vi "pco.camera_SaveMean_Example_IMAQ.vi"() -> ()   [LabVIEW 2020]
uses:
  Camera.lvclass
panel:
  out "rawImage":u16[][](array[numeric])
  out "Image":T1(plugin-control)
  in  "data_format":T2(ring)=enum."Mono16"
  in  "Image Index":u32 max=9
  in  "saveImages":bool
  in  "SavePath":path
  out "Recorded Images":u32
  in  "Quit":bool
  in  "roiY1":u64=2 min=2 max=1040 step=1
  in  "roiX1":u64=2 min=2 max=1392 step=1
  in  "roiY0":u64=1 min=1 max=1039 step=1
  in  "roiX0":u64=1 min=1 max=1391 step=1
  out "Image Height":u16
  out "Image Width":u16
  in  "dwImgCount":u32=10 caption="Required Number of Images" max=4023
  out "Error":errorcluster {"code" format="%x"}
  # "This example shows how to record an image sequence, get the mean of that sequence and save it to file afterwards.\nIt is a good starting point for writing own applications.\nBut it will not be fail save, i.e. doesnt react on errors, just handles them forward to the end\n\nUsage:\nSelect your required image count you want to average over before you start the program.\nOnce started, the camera class will be initialized and images will be recorded automatically.\nTWhen acquisition has finished the mean image is read and shown.\nNow you can crop the image using the ROI parameters and select a file path.\nBy clicking save, the mean image is saved with the selected file format using the current roi setting\nThis also finishes the program and will force an exit of the camera class"
  # "pco.labview"
  # "Camera Setup"
  # "Recording Control"
  # "Parameters for image readout"
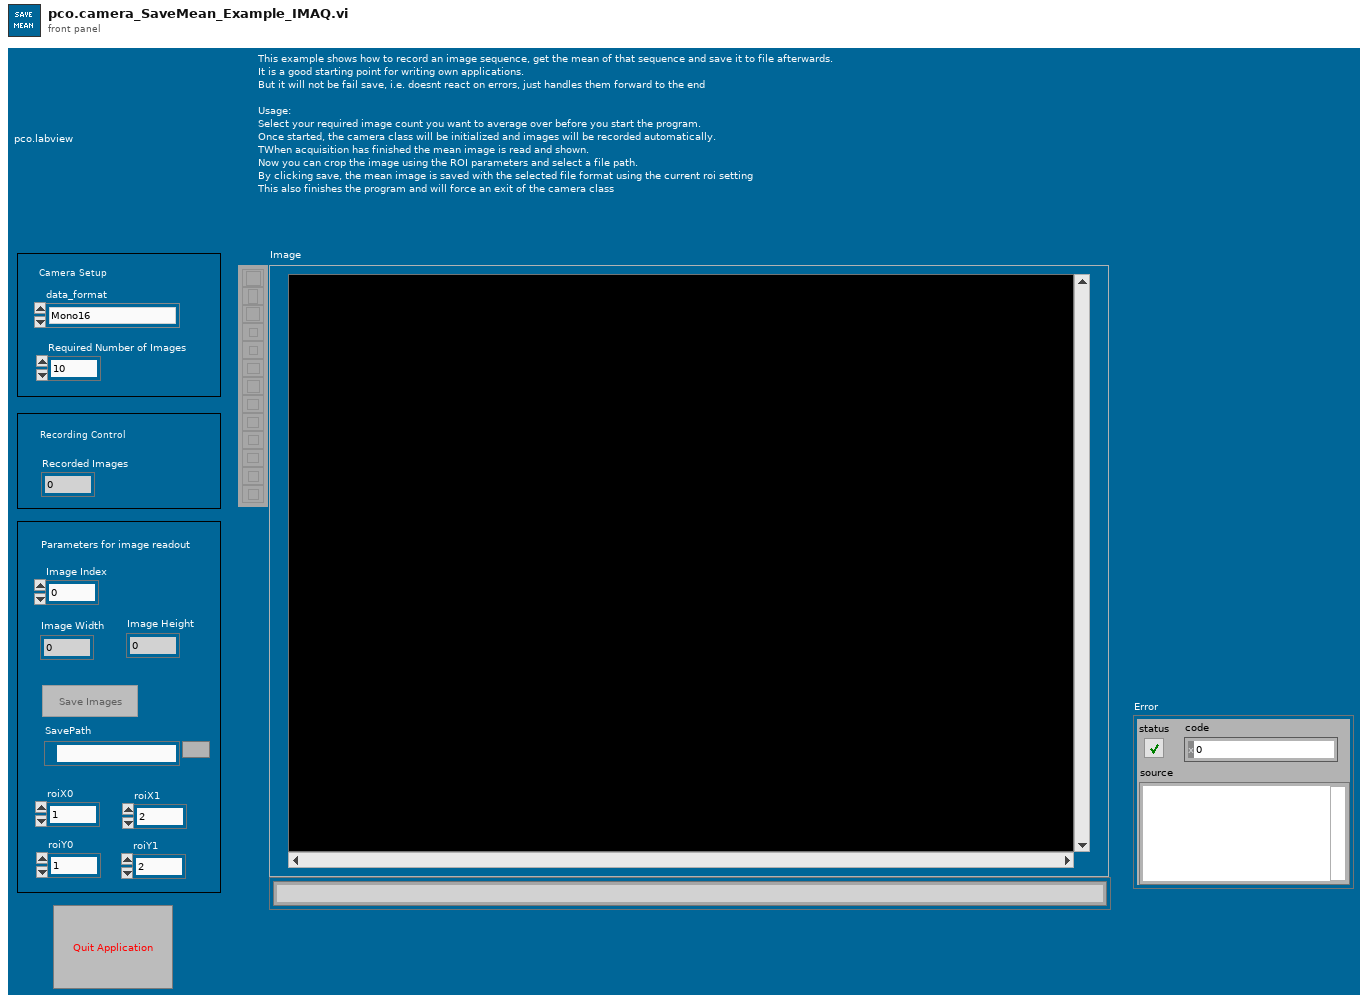
[diagram p1: front panel]
types:
  T1 = typedef "IMAQ Image.ctl" = refnum<image>
  T2 = enum16{"Undefined", "Mono8", "Mono16", "BGRA8", "RGBA8", "BGRA16", "RGBA16", "CompressedMono8"}
  T3 = enum8{"Enabled", "Disabled", "Disabled and Grayed Out"}
  T4 = enum16{"sequence", "sequence non blocking", "ring buffer", "fifo", "sequence_dpcore", "sequence_non_blocking_dpcore", "ring_buffer_dpcore", "fifo_dpcore", "tif", "multitif", "pcoraw", "b16", "dicom", "multidicom"}
  T5 = cluster{"serial":u32, "type":u16, "sub_type":u16, "interface_type":u16, "bit_resolution":u16, "min_exposure_time_s":dbl, "max_exposure_time_s":dbl, "min_exposure_step_s":dbl, "min_delay_time_s":dbl, "max_delay_time_s":dbl, "min_delay_step_s":dbl, "min_width":u64, "min_height":u64, "max_width":u64, "max_height":u64, "roi_step_horz":u64, "roi_step_vert":u64, "roi_symmetric_horz":bool, "roi_symmetric_vert":bool, "has_timestamp_mode":bool, "has_timestamp_mode_ascii_only":bool, "pixelrate_vec":u32[], "has_acquire_mode":bool, "has_ext_acquire_mode":bool, "has_metadata_mode":bool, "has_ram":bool, "binning_horz_vec":u16[], "binning_vert_vec":u16[]}
  T6 = typedef "Image Type" = u32
  T7 = typedef "Camera.lvclass/binning.ctl" = cluster{"vert":u16, "horz":u16}
  T8 = cluster{"exposure_time_s":dbl, "delay_time_s":dbl, "roi":cluster{"x0":u64, "y0":u64, "x1":u64, "y1":u64}, "timestamp_mode":u16, "pixelrate":u32, "trigger_mode":u16, "acquire_mode":u16, "metadata_mode":u16, "noisefilter_mode":u16, "binning":T7}
  T9 = cluster{"Plane 4 (alpha)":u16, "Plane 1 (Red)":u16, "Plane 2 (Green)":u16, "Plane 3 (Blue)":u16}[][]
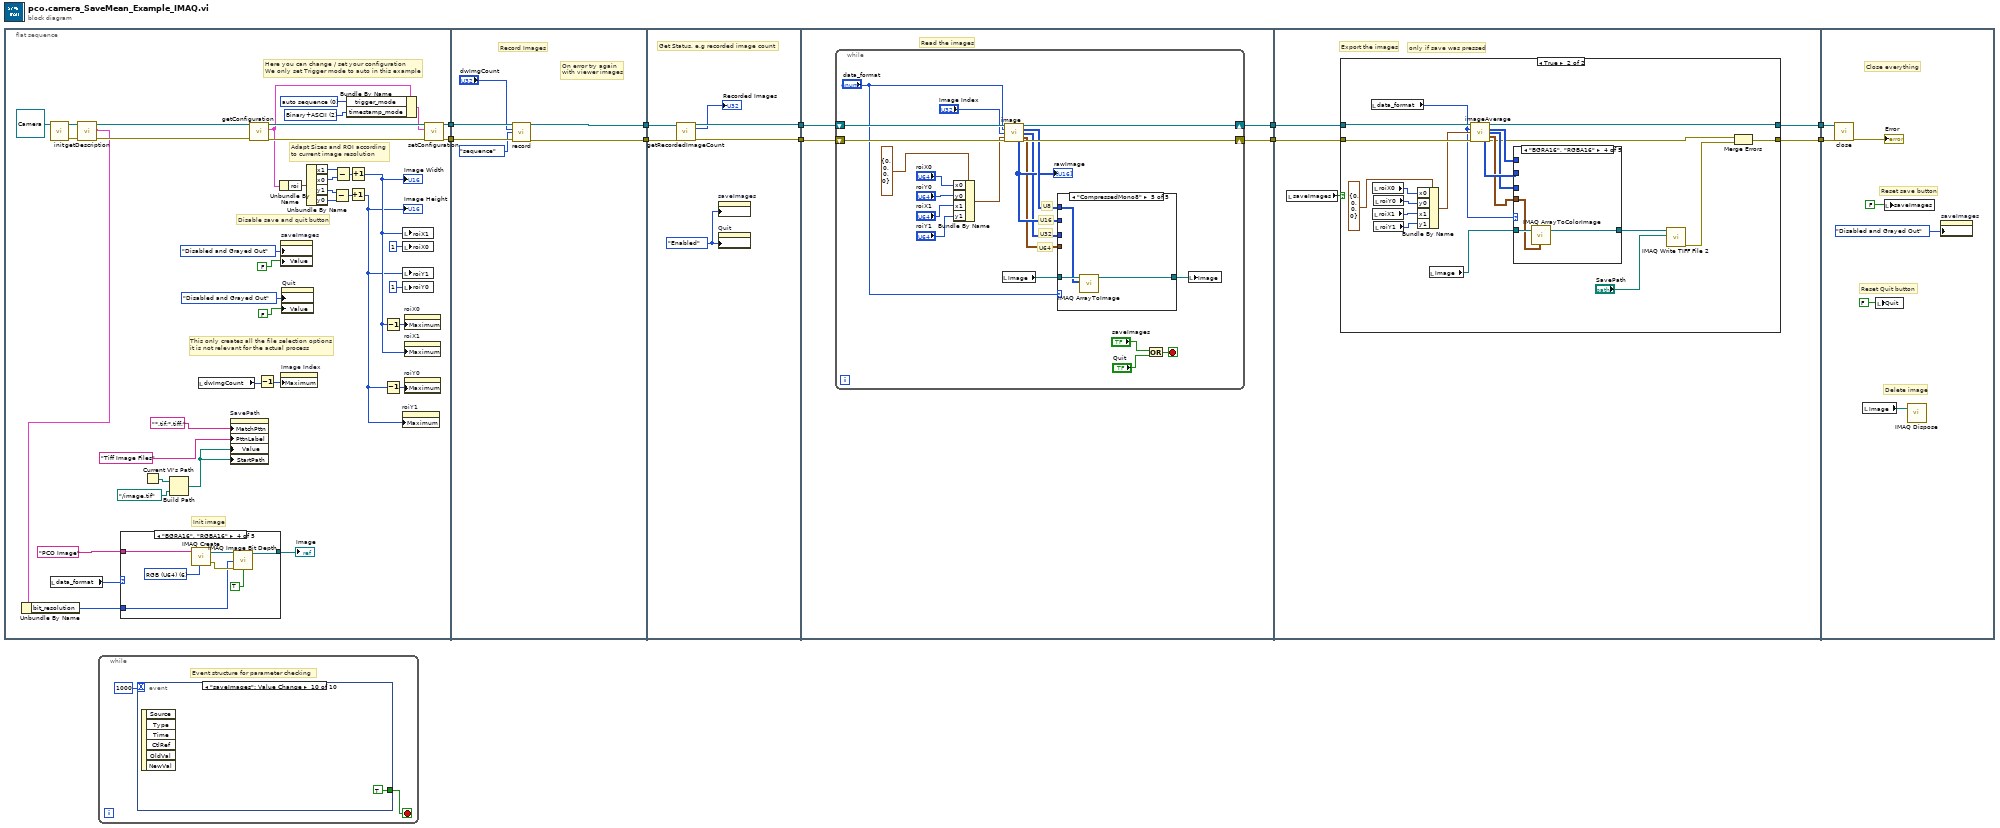
[diagram p0: block diagram]
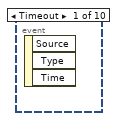
[diagram p2: hidden frame]
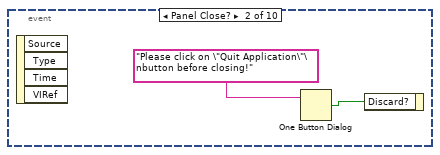
[diagram p3: hidden frame]
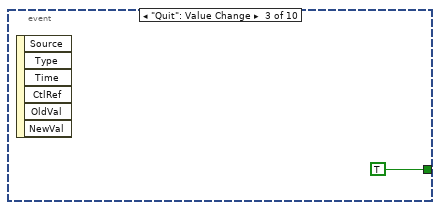
[diagram p4: hidden frame]
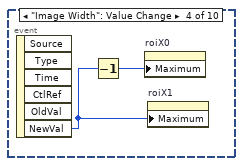
[diagram p5: hidden frame]
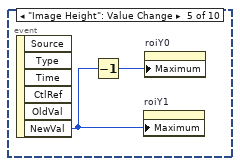
[diagram p6: hidden frame]
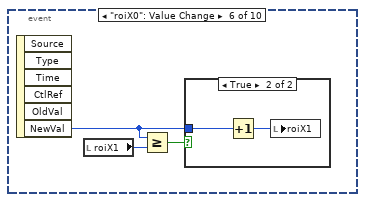
[diagram p7: hidden frame]
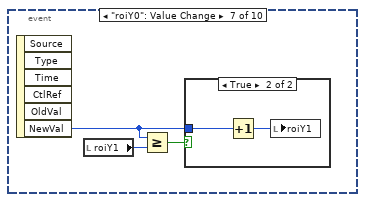
[diagram p9: hidden frame]
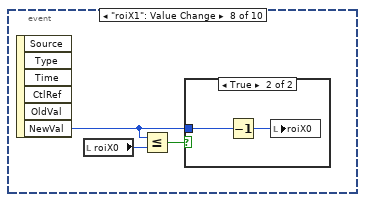
[diagram p11: hidden frame]
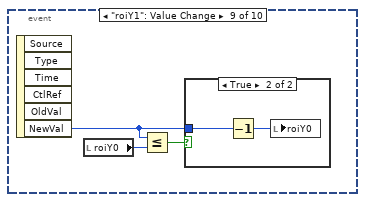
[diagram p13: hidden frame]
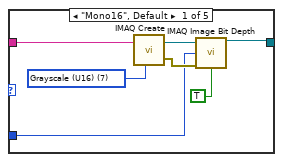
[diagram p15: hidden frame]
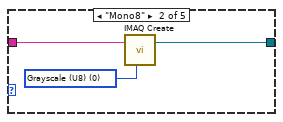
[diagram p16: hidden frame]
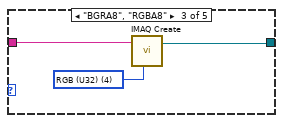
[diagram p17: hidden frame]
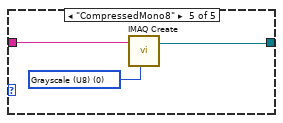
[diagram p18: hidden frame]
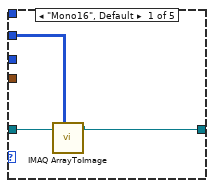
[diagram p19: hidden frame]
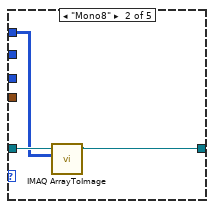
[diagram p20: hidden frame]
diagram:
  n1 = flat-sequence {
    tunnel: [w45] -> w10
    tunnel: [w44] -> w9
    tunnel: w10 -> [w81]
    tunnel: w9 -> [w80]
    tunnel: [w78] -> w8
    tunnel: [w77] -> w7
    tunnel: w8 -> [w87]
    tunnel: w7 -> [w86]
    tunnel: [w85] -> w6
    tunnel: [w84] -> w5
    tunnel: w6 -> [w90]
    tunnel: w5 -> [w91]
    tunnel: [w89] -> w4
    tunnel: [w88] -> w2
    tunnel: w4 -> [w131]
    tunnel: [w130] -> w3
    tunnel: w2 -> [w129]
    tunnel: [w128] -> w1
    tunnel: w3 -> [w176]
    tunnel: w1 -> [w175]
    frame #0 {
      w29 = u16 2 items=["OFF", "Binary", "Binary+ASCII", "ASCII"] ("TimestampMode")
      w51 = u16 0 items=["auto sequence"=0, "software trigger"=1, "external exposure start & software trigger"=2, "external exposure control"=3, "external synchronized"=4, "fast external exposure control"=5, "external CDS control"=6, "slow external exposure control"=7, "external synchronized HDSDI"=258] ("TriggerMode")
      # "Init image"
      # "This only creates all the file selection options\nit is not relevant for the actual process"
      # "Adapt Sizes and ROI according\nto current image resolution"
      # "Disable save and quit button"
      # "Here you can change / set your configuration\nWe only set Trigger mode to auto in this example"
      n2 = call-dynamic "init.vi"("Camera in"=refnum<class "Camera.lvclass"> refnum ("PCOCamera in")) -> ("Camera out"=w15:refnum<class "Camera.lvclass">, "error out"=w16:errorcluster)  [unwired: 8 in]
      n3 = local read "data_format"() -> (w19:T2)
      n4 = call-dynamic "getDescription.vi"("error in (no error)"=w16, "Camera in"=w15) -> ("error out"=w13:errorcluster, "description"=w12:T5, "Camera out"=w14:refnum<class "Camera.lvclass">)  [unwired: 7 in]
      n5 = Unbundle By Name(w12) -> ("bit_resolution"=w11:u16)
      n6 = case shown="\"BGRA16\", \"RGBA16\"" w19 {
        tunnel: "PCO Image" ("Image Name") -> [w58 w62 w64 w71 w74]
        tunnel: [w54 w60 w63 w68 w73] -> w18
        tunnel: w11 -> [w53 _ _ w66 _]
        frame "Mono16", Default {
          w59 = T6 7 items=["Grayscale (U8)", "Grayscale (I16)", "Grayscale (SGL)", "Complex (CSG)", "RGB (U32)", "HSL (U32)", "RGB (U64)", "Grayscale (U16)"] ("Image Type")
          n7 = call "IMAQ Create"("Image Name"=w58, "Image Type"=w59) -> ("New Image"=w56:T1, "error out"=w55:errorcluster)  [unwired: 3 in]
          n8 = call "IMAQ Image Bit Depth"("Image"=w56, "Bit Depth (0)"=w53, "error in (no error)"=w55, "Get/Set Bit Depth? (Set)"=TRUE) -> ("Image Out"=w54:T1)  [unwired: 9 in, 2 out]
        }
        frame "Mono8" {
          w61 = T6 0 items=["Grayscale (U8)", "Grayscale (I16)", "Grayscale (SGL)", "Complex (CSG)", "RGB (U32)", "HSL (U32)", "RGB (U64)", "Grayscale (U16)"] ("Image Type")
          n9 = call "IMAQ Create"("Image Name"=w62, "Image Type"=w61) -> ("New Image"=w60:T1)  [unwired: 3 in, 1 out]
        }
        frame "BGRA8", "RGBA8" {
          w65 = T6 4 items=["Grayscale (U8)", "Grayscale (I16)", "Grayscale (SGL)", "Complex (CSG)", "RGB (U32)", "HSL (U32)", "RGB (U64)", "Grayscale (U16)"] ("Image Type")
          n10 = call "IMAQ Create"("Image Name"=w64, "Image Type"=w65) -> ("New Image"=w63:T1)  [unwired: 3 in, 1 out]
        }
        frame "BGRA16", "RGBA16" {
          w72 = T6 6 items=["Grayscale (U8)", "Grayscale (I16)", "Grayscale (SGL)", "Complex (CSG)", "RGB (U32)", "HSL (U32)", "RGB (U64)", "Grayscale (U16)"] ("Image Type")
          n11 = call "IMAQ Create"("Image Name"=w71, "Image Type"=w72) -> ("New Image"=w69:T1, "error out"=w67:errorcluster)  [unwired: 3 in]
          n12 = call "IMAQ Image Bit Depth"("Image"=w69, "Bit Depth (0)"=w66, "error in (no error)"=w67, "Get/Set Bit Depth? (Set)"=TRUE) -> ("Image Out"=w68:T1)  [unwired: 9 in, 2 out]
        }
        frame "CompressedMono8" {
          w75 = T6 0 items=["Grayscale (U8)", "Grayscale (I16)", "Grayscale (SGL)", "Complex (CSG)", "RGB (U32)", "HSL (U32)", "RGB (U64)", "Grayscale (U16)"] ("Image Type")
          n13 = call "IMAQ Create"("Image Name"=w74, "Image Type"=w75) -> ("New Image"=w73:T1)  [unwired: 3 in, 1 out]
        }
      }
      "Image" <- w18
      n14 = Current VI's Path() -> (path=w26:path)
      n15 = Build Path(base path=w26, name or relative path=path "../image.tif" ("SavePath")) -> (appended path=w23:path)
      n16 = local read "dwImgCount"() -> (w21:u32)
      n17 = property on="SavePath" class="Path"("MatchPttn"="*.tif;*.tiff;" ("pattern (all files)"), "PttnLabel"="Tiff Image Files" ("pattern label"), "Value"=w23, "StartPath"=w23) -> ()  [unwired: 2 in, 2 out]
      n18 = call-dynamic "getConfiguration.vi"("error in (no error)"=w13, "Camera in"=w14) -> ("error out"=w49:errorcluster, "configuration"=w39:T8, "Camera out"=w50:refnum<class "Camera.lvclass">)  [unwired: 7 in]
      n19 = Decrement(x=w21) -> (x-1=w22:u32)
      n20 = Unbundle By Name(w39) -> ("roi"=w38:cluster{"x0":u64, "y0":u64, "x1":u64, "y1":u64})
      n21 = property on="saveImages" class="Bool (strict)"("DisabledEnum"=T3."Disabled and Grayed Out" ("Disabled"), "Value"=FALSE ("Stop")) -> ()  [unwired: 2 in, 2 out]
      n22 = property on="Image Index" class="DigNum (strict)"("Maximum"=w22) -> ()  [unwired: 2 in, 2 out]
      n23 = property on="Quit" class="Bool (strict)"("DisabledEnum"=T3."Disabled and Grayed Out" ("Disabled"), "Value"=FALSE ("Stop")) -> ()  [unwired: 2 in, 2 out]
      n24 = Unbundle By Name(w38) -> ("x1"=w36:u64, "x0"=w37:u64, "y1"=w34:u64, "y0"=w35:u64)
      n25 = Subtract(x=w34, y=w35) -> (x-y=w32:u64)
      n26 = Subtract(x=w36, y=w37) -> (x-y=w33:u64)
      n27 = Bundle By Name(cluster=w39, "trigger_mode"=w51, "timestamp_mode"=w29) -> (w48:T8)
      n28 = Increment(x=w32) -> (x+1=w30:u64)
      "Image Height" <- w30
      n29 = Increment(x=w33) -> (x+1=w31:u64)
      "Image Width" <- w31
      n30 = Decrement(x=w31) -> (x-1=w41:u64)
      n31 = Decrement(x=w30) -> (x-1=w40:u64)
      n32 = property on="roiY1" class="DigNum (strict)"("Maximum"=w30) -> ()  [unwired: 2 in, 2 out]
      n33 = local write "roiX1"(w31) -> ()
      n34 = local write "roiX0"(u16 1 ("roiY0")) -> ()
      n35 = local write "roiY1"(w30) -> ()
      n36 = local write "roiY0"(u16 1 ("roiY0")) -> ()
      n37 = property on="roiX0" class="DigNum (strict)"("Maximum"=w41) -> ()  [unwired: 2 in, 2 out]
      n38 = property on="roiX1" class="DigNum (strict)"("Maximum"=w31) -> ()  [unwired: 2 in, 2 out]
      n39 = property on="roiY0" class="DigNum (strict)"("Maximum"=w40) -> ()  [unwired: 2 in, 2 out]
      n40 = call-dynamic "setConfiguration.vi"("error in (no error)"=w49, "configuration"=w48, "Camera in"=w50) -> ("error out"=w44:errorcluster, "Camera out"=w45:refnum<class "Camera.lvclass">)  [unwired: 7 in]
    }
    frame #1 {
      # "On error try again \nwith viewer images"
      # "Record Images"
      n41 = call-dynamic "record.vi"("Camera in"=w81, "num_images"="dwImgCount", "record_mode"=T4."sequence", "error in (no error)"=w80) -> ("Camera out"=w78:refnum<class "Camera.lvclass">, "error out"=w77:errorcluster)  [unwired: 10 in]
    }
    frame #2 {
      w82 = T3."Enabled" ("Disabled")
      # "Get Status, e.g recorded image count"
      n42 = call-dynamic "getRecordedImageCount.vi"("Camera in"=w87, "error in (no error)"=w86) -> ("Camera out"=w85:refnum<class "Camera.lvclass">, "recorded_image_count"=→"Recorded Images":u32, "error out"=w84:errorcluster)  [unwired: 11 in]
      n43 = property on="saveImages" class="Bool (strict)"("DisabledEnum"=w82) -> ()  [unwired: 2 in, 2 out]
      n44 = property on="Quit" class="Bool (strict)"("DisabledEnum"=w82) -> ()  [unwired: 2 in, 2 out]
    }
    frame #3 {
      # "Read the images"
      n45 = while {
        shift-right: [w110] -> w89
        shift-left: w90 -> [w112]
        shift-right: [w105] -> w88
        shift-left: w91 -> [w111]
        stop <- w103 stop-if-true
        # "U64"
        # "U32"
        # "U16"
        # "U8"
        n46 = Bundle By Name(cluster=cluster{"x0":u64, "y0":u64, "x1":u64, "y1":u64} {"x0"=0, "y0"=0, "x1"=0, "y1"=0} ("roi"), "x0"="roiX0", "y0"="roiY0", "x1"="roiX1", "y1"="roiY1") -> (w101:cluster{"x0":u64, "y0":u64, "x1":u64, "y1":u64})
        n47 = local read "Image"() -> (w94:T1)
        n48 = call-dynamic "image.vi"("Camera in"=w112, "data_format"="data_format", "image_index"="Image Index", "roi"=w101, "error in (no error)"=w111) -> ("Camera out"=w110:refnum<class "Camera.lvclass">, "image (U8)"=w98:u8[][], "image (U32)"=w96:u32[][], "image (U64)"=w95:T9, "raw_image (U16)"=w97:u16[][], "error out"=w105:errorcluster)  [unwired: 3 in, 2 out]
        "rawImage" <- w97
        n49 = case shown="\"CompressedMono8\"" "data_format" {
          tunnel: w94 -> [w115 w118 w121 w124 w127]
          tunnel: [w113 w116 w120 w122 w126] -> w93
          tunnel: w95 -> [_ _ _ w123 _]
          tunnel: w96 -> [_ _ w119 _ _]
          tunnel: w98 -> [_ w117 _ _ w125]
          tunnel: w97 -> [w114 _ _ _ _]
          frame "Mono16", Default {
            n50 = call "IMAQ ArrayToImage"("Image Pixels (U16)"=w114, "Image"=w115) -> ("Image Out"=w113:T1)  [unwired: 8 in, 1 out]
          }
          frame "Mono8" {
            n51 = call "IMAQ ArrayToImage"("Image Pixels (U8)"=w117, "Image"=w118) -> ("Image Out"=w116:T1)  [unwired: 8 in, 1 out]
          }
          frame "BGRA8", "RGBA8" {
            n52 = call "IMAQ ArrayToColorImage"("Image Pixels (U32)"=w119, "Image"=w121) -> ("Image Out"=w120:T1)  [unwired: 3 in, 1 out]
          }
          frame "BGRA16", "RGBA16" {
            n53 = call "IMAQ ArrayToColorImage"("Image"=w124, "Image Pixels (U64)"=w123) -> ("Image Out"=w122:T1)  [unwired: 3 in, 1 out]
          }
          frame "CompressedMono8" {
            n54 = call "IMAQ ArrayToImage"("Image Pixels (U8)"=w125, "Image"=w127) -> ("Image Out"=w126:T1)  [unwired: 8 in, 1 out]
          }
        }
        n55 = Or(x="saveImages", y="Quit") -> (x .or. y?=w103:bool)
        n56 = local write "Image"(w93) -> ()
      }
    }
    frame #4 {
      # "only if save was pressed"
      # "Export the images"
      n57 = local read "saveImages"() -> (w132:bool)
      n58 = case shown="True" w132 {
        tunnel: w131 -> [w134 w153]
        tunnel: [w134 w142] -> w130
        tunnel: w129 -> [w133 w154]
        tunnel: [w133 w140] -> w128
        frame False {
        }
        frame True {
          n59 = local read "data_format"() -> (w138:T2)
          n60 = local read "roiX0"() -> (w151:u64)
          n61 = local read "roiX1"() -> (w149:u64)
          n62 = local read "roiY0"() -> (w150:u64)
          n63 = local read "roiY1"() -> (w148:u64)
          n64 = Bundle By Name(cluster=cluster{"x0":u64, "y0":u64, "x1":u64, "y1":u64} {"x0"=0, "y0"=0, "x1"=0, "y1"=0} ("roi"), "x0"=w151, "y0"=w150, "x1"=w149, "y1"=w148) -> (w147:cluster{"x0":u64, "y0":u64, "x1":u64, "y1":u64})
          n65 = local read "Image"() -> (w139:T1)
          n66 = call-dynamic "imageAverage.vi"("Camera in"=w153, "data_format"=w138, "roi"=w147, "error in (no error)"=w154) -> ("Camera out"=w142:refnum<class "Camera.lvclass">, "image (U8)"=w146:u8[][], "image (U32)"=w144:u32[][], "image (U64)"=w143:T9, "raw_image (U16)"=w145:u16[][], "error out"=w141:errorcluster)  [unwired: 6 in]
          n67 = case shown="\"BGRA16\", \"RGBA16\"" w138 {
            tunnel: w139 -> [w157 w160 w163 w166 w169]
            tunnel: [w155 w158 w162 w164 w168] -> w136
            tunnel: w143 -> [_ _ _ w165 _]
            tunnel: w144 -> [_ _ w161 _ _]
            tunnel: w146 -> [_ w159 _ _ w167]
            tunnel: w145 -> [w156 _ _ _ _]
            frame "Mono16", Default {
              n68 = call "IMAQ ArrayToImage"("Image Pixels (U16)"=w156, "Image"=w157) -> ("Image Out"=w155:T1)  [unwired: 8 in, 1 out]
            }
            frame "Mono8" {
              n69 = call "IMAQ ArrayToImage"("Image Pixels (U8)"=w159, "Image"=w160) -> ("Image Out"=w158:T1)  [unwired: 8 in, 1 out]
            }
            frame "BGRA8", "RGBA8" {
              n70 = call "IMAQ ArrayToColorImage"("Image Pixels (U32)"=w161, "Image"=w163) -> ("Image Out"=w162:T1)  [unwired: 3 in, 1 out]
            }
            frame "BGRA16", "RGBA16" {
              n71 = call "IMAQ ArrayToColorImage"("Image"=w166, "Image Pixels (U64)"=w165) -> ("Image Out"=w164:T1)  [unwired: 3 in, 1 out]
            }
            frame "CompressedMono8" {
              n72 = call "IMAQ ArrayToImage"("Image Pixels (U8)"=w167, "Image"=w169) -> ("Image Out"=w168:T1)  [unwired: 8 in, 1 out]
            }
          }
          n73 = call "IMAQ Write TIFF File 2"("File Path"="SavePath", "Image"=w136) -> ("error out"=w137:errorcluster)  [unwired: 8 in, 1 out]
          n74 = Merge Errors(w141, w137) -> (w140:errorcluster)
        }
      }
    }
    frame #5 {
      # "Delete image"
      # "Reset Quit button"
      # "Close everything"
      # "Reset save button"
      n75 = call-dynamic "close.vi"("error in (no error)"=w175, "Camera in"=w176) -> ("error out"=→"Error":errorcluster)  [unwired: 9 in]
      n76 = local read "Image"() -> (w170:T1)
      n77 = local write "Quit"(FALSE ("Stop")) -> ()
      n78 = local write "saveImages"(FALSE ("Stop")) -> ()
      n79 = call "IMAQ Dispose"("Image"=w170) -> ()  [unwired: 5 in, 1 out]
      n80 = property on="saveImages" class="Bool (strict)"("DisabledEnum"=T3."Disabled and Grayed Out" ("Disabled")) -> ()  [unwired: 2 in, 2 out]
    }
  }
  n81 = while {
    stop <- w177 stop-if-true
    # "Event structure for parameter checking"
    n82 = event shown="[9] \"saveImages\": Value Change" {
      selector: _ -> [_ _ _ _ _ _ _ _ _ _]
      dyn-events: _ -> [_ _ _ _ _ _ _ _ _ _]
      timeout: 1000 -> [_ _ _ _ _ _ _ _ _ _]
      tunnel: [_ _ TRUE _ _ _ _ _ _ TRUE] -> w177
      event Timeout {
        n83 = event-data() -> ()  [unwired: 1 in, 3 out]
      }
      event Panel Close? {
        n84 = event-data() -> ()  [unwired: 1 in, 4 out]
        n85 = One Button Dialog(message="Please click on \"Quit Application\"\nbutton before closing!") -> (true=w179:bool)  [unwired: 1 in]
        n86 = event-data("Discard?"=w179) -> ()  [unwired: 1 in, 1 out]
      }
      event "Quit": Value Change {
        n87 = event-data() -> ()  [unwired: 1 in, 6 out]
      }
      event "Image Width": Value Change {
        n88 = event-data() -> ("NewVal"=w182:u16)  [unwired: 1 in, 5 out]
        n89 = Decrement(x=w182) -> (x-1=w183:u16)
        n90 = property on="roiX0" class="DigNum (strict)"("Maximum"=w183) -> ()  [unwired: 2 in, 2 out]
        n91 = property on="roiX1" class="DigNum (strict)"("Maximum"=w182) -> ()  [unwired: 2 in, 2 out]
      }
      event "Image Height": Value Change {
        n92 = event-data() -> ("NewVal"=w184:u16)  [unwired: 1 in, 5 out]
        n93 = Decrement(x=w184) -> (x-1=w185:u16)
        n94 = property on="roiY1" class="DigNum (strict)"("Maximum"=w184) -> ()  [unwired: 2 in, 2 out]
        n95 = property on="roiY0" class="DigNum (strict)"("Maximum"=w185) -> ()  [unwired: 2 in, 2 out]
      }
      event "roiX0": Value Change {
        n96 = event-data() -> ("NewVal"=w186:u64)  [unwired: 1 in, 5 out]
        n97 = local read "roiX1"() -> (w188:u64)
        n98 = Greater Or Equal?(x=w186, y=w188) -> (x >= y?=w187:bool)
        n99 = case shown="True" w187 {
          tunnel: w186 -> [_ w190]
          frame False {
          }
          frame True {
            n100 = Increment(x=w190) -> (x+1=w189:u64)
            n101 = local write "roiX1"(w189) -> ()
          }
        }
      }
      event "roiY0": Value Change {
        n102 = event-data() -> ("NewVal"=w191:u64)  [unwired: 1 in, 5 out]
        n103 = local read "roiY1"() -> (w193:u64)
        n104 = Greater Or Equal?(x=w191, y=w193) -> (x >= y?=w192:bool)
        n105 = case shown="True" w192 {
          tunnel: w191 -> [_ w195]
          frame False {
          }
          frame True {
            n106 = Increment(x=w195) -> (x+1=w194:u64)
            n107 = local write "roiY1"(w194) -> ()
          }
        }
      }
      event "roiX1": Value Change {
        n108 = event-data() -> ("NewVal"=w196:u64)  [unwired: 1 in, 5 out]
        n109 = local read "roiX0"() -> (w198:u64)
        n110 = Less Or Equal?(x=w196, y=w198) -> (x <= y?=w197:bool)
        n111 = case shown="True" w197 {
          tunnel: w196 -> [_ w200]
          frame False {
          }
          frame True {
            n112 = Decrement(x=w200) -> (x-1=w199:u64)
            n113 = local write "roiX0"(w199) -> ()
          }
        }
      }
      event "roiY1": Value Change {
        n114 = event-data() -> ("NewVal"=w201:u64)  [unwired: 1 in, 5 out]
        n115 = local read "roiY0"() -> (w203:u64)
        n116 = Less Or Equal?(x=w201, y=w203) -> (x <= y?=w202:bool)
        n117 = case shown="True" w202 {
          tunnel: w201 -> [_ w205]
          frame False {
          }
          frame True {
            n118 = Decrement(x=w205) -> (x-1=w204:u64)
            n119 = local write "roiY0"(w204) -> ()
          }
        }
      }
      event "saveImages": Value Change {
        n120 = event-data() -> ()  [unwired: 1 in, 6 out]
      }
    }
  }
